vi "Initialize Log File.vi"(8 "error in (no error)":errorcluster, 9 "Operation":T1, 10 "File Path":path, 11 "Log File Specification in":refnum<class "Log File Specification.lvclass">) -> (0 "error out":errorcluster, 1 "Log File out":refnum<class "Log File.lvclass">, 3 "Log File Specification out":refnum<class "Log File Specification.lvclass">)   [LabVIEW 2015, in "Log File Specification.lvclass"]
uses:
  Log File Specification.lvclass
  Logs/Log Files/Log File/Log File.lvclass
  Logs/Log Files/Log File/Operation.ctl
  Log File Specification.lvclass/Log File Specification.ctl
  TDMS Log File Specification/TDMS Log File Specification.lvclass
  Waveform TDMS Log File Specification/Waveform TDMS Log File Specification.lvclass
  Text Log File Specification/Text Log File Specification.lvclass
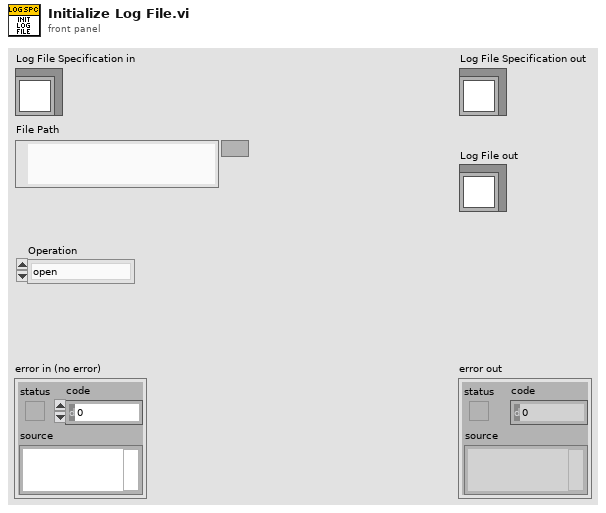
[diagram p1: front panel]
types:
  T1 = typedef "Log File.lvclass/Operation.ctl" = enum16{"open", "open or create", "create or replace", "create", "open (read-only)"}
  T2 = typedef "Log File Specification.lvclass/Log Specification Type.ctl" = enum16{"Default", "TDMS", "Text", "Waveform TDMS"}
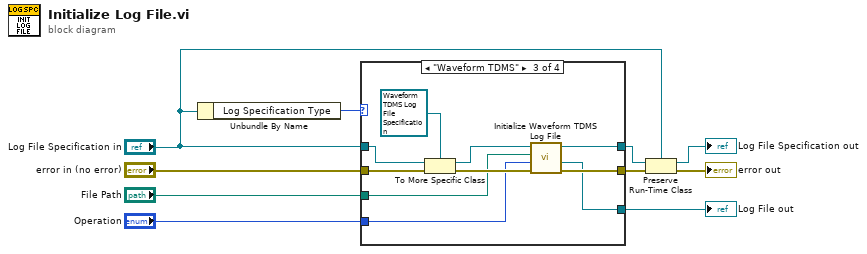
[diagram p0: block diagram]
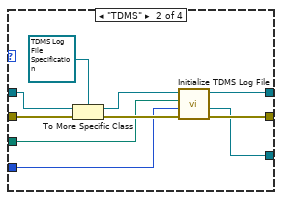
[diagram p3: hidden frame]
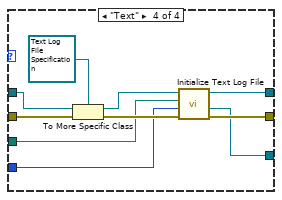
[diagram p4: hidden frame]
diagram:
  n1 = Unbundle By Name("Log File Specification in") -> ("Log Specification Type"=w10:T2)
  n2 = case shown="\"Waveform TDMS\"" w10 {
    tunnel: "error in (no error)" -> [w11 w22 w32 w42]
    tunnel: "Log File Specification in" -> [w12 w19 w29 w39]
    tunnel: [w12 w18 w28 w38] -> w2
    tunnel: [w11 w16 w26 w36] -> w5
    tunnel: "File Path" -> [_ w15 w25 w35]
    tunnel: "Operation" -> [_ w14 w24 w34]
    tunnel: [_ w13 w23 w33] -> w6
    frame "Default", Default {
    }
    frame "TDMS" {
      n3 = To More Specific Class(target class=refnum<class "TDMS Log File Specification.lvclass"> refnum ("TDMS Log File Specification.lvclass"), reference=w19, error in=w22) -> (specific class reference=w17:refnum<class "TDMS Log File Specification.lvclass">, error out=w21:errorcluster)
      n4 = call "Initialize TDMS Log File.vi"("error in (no error)"=w21, "Operation"=w14, "File Path"=w15, "TDMS Log File Specification in"=w17) -> ("error out"=w16:errorcluster, "Log File out"=w13:refnum<class "Log File.lvclass">, "TDMS Log File Specification out"=w18:refnum<class "TDMS Log File Specification.lvclass">)  [unwired: 5 in]
    }
    frame "Waveform TDMS" {
      n5 = To More Specific Class(target class=refnum<class "Waveform TDMS Log File Specification.lvclass"> refnum ("TDMS Log File Specification.lvclass"), reference=w29, error in=w32) -> (specific class reference=w27:refnum<class "Waveform TDMS Log File Specification.lvclass">, error out=w31:errorcluster)
      n6 = call "Initialize Waveform TDMS Log File.vi"("error in (no error)"=w31, "Operation"=w24, "File Path"=w25, "Waveform TDMS Log File Specification in"=w27) -> ("error out"=w26:errorcluster, "Log File out"=w23:refnum<class "Log File.lvclass">, "Waveform TDMS Log File Specification out"=w28:refnum<class "Waveform TDMS Log File Specification.lvclass">)  [unwired: 5 in]
    }
    frame "Text" {
      n7 = To More Specific Class(target class=refnum<class "Text Log File Specification.lvclass"> refnum ("Text Log File Specification.lvclass"), reference=w39, error in=w42) -> (specific class reference=w37:refnum<class "Text Log File Specification.lvclass">, error out=w41:errorcluster)
      n8 = call "Initialize Text Log File.vi"("error in (no error)"=w41, "Operation"=w34, "File Path"=w35, "Text Log File Specification in"=w37) -> ("error out"=w36:errorcluster, "Log File out"=w33:refnum<class "Log File.lvclass">, "Text Log File Specification out"=w38:refnum<class "Text Log File Specification.lvclass">)  [unwired: 5 in]
    }
  }
  "Log File out" <- w6
  n9 = Preserve Run-Time Class(object in=w2, error in=w5, 2:"Log File Specification in") -> (object out=→"Log File Specification out":refnum<class "Log File Specification.lvclass">, error out=→"error out":errorcluster)
